vi "readParameterFromXML.vi"(8 "error in (no error)":errorcluster, 10 "eventXML":refnum<k20>, 11 "ScriptEvent in":refnum<class "ScriptEvent.lvclass">) -> (0 "error out":errorcluster, 2 "eventXML out":refnum<k20>, 3 "ScriptEvent out":refnum<class "ScriptEvent.lvclass">)   [LabVIEW 2009, in "Tools.lvlib" / "Scripting.lvlib" / "ScriptEvent.lvclass"]
uses:
  ScriptEvent.lvclass
  <vilib>/xml/Close Reference(Node).vi
  ScriptEvent.lvclass/ScriptEvent.ctl
  <vilib>/xml/NI_XML.lvlib
  Program Files/National Instruments/LabVIEW 2009/resource/objmgr/DOMUserDefRef.rc
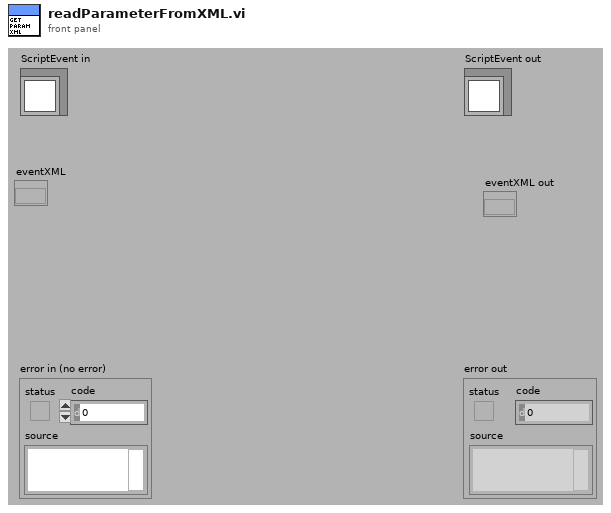
[diagram p1: front panel]
types:
  T1 = cluster{"parameter_name":string, "parameter_value":string, "type":enum16{"time", "time_difference", "value", "frequency", "phase", "ramp_time", "value_step", "time_step", "number_of_steps", "start_value", "end_value", "start_freq", "start_amp", "start_phase", "end_freq", "end_amp", "end_phase"}}
  T2 = enum16{"time", "time_difference", "value", "frequency", "phase", "ramp_time", "value_step", "time_step", "number_of_steps", "start_value", "end_value", "start_freq", "start_amp", "start_phase", "end_freq", "end_amp", "end_phase"}
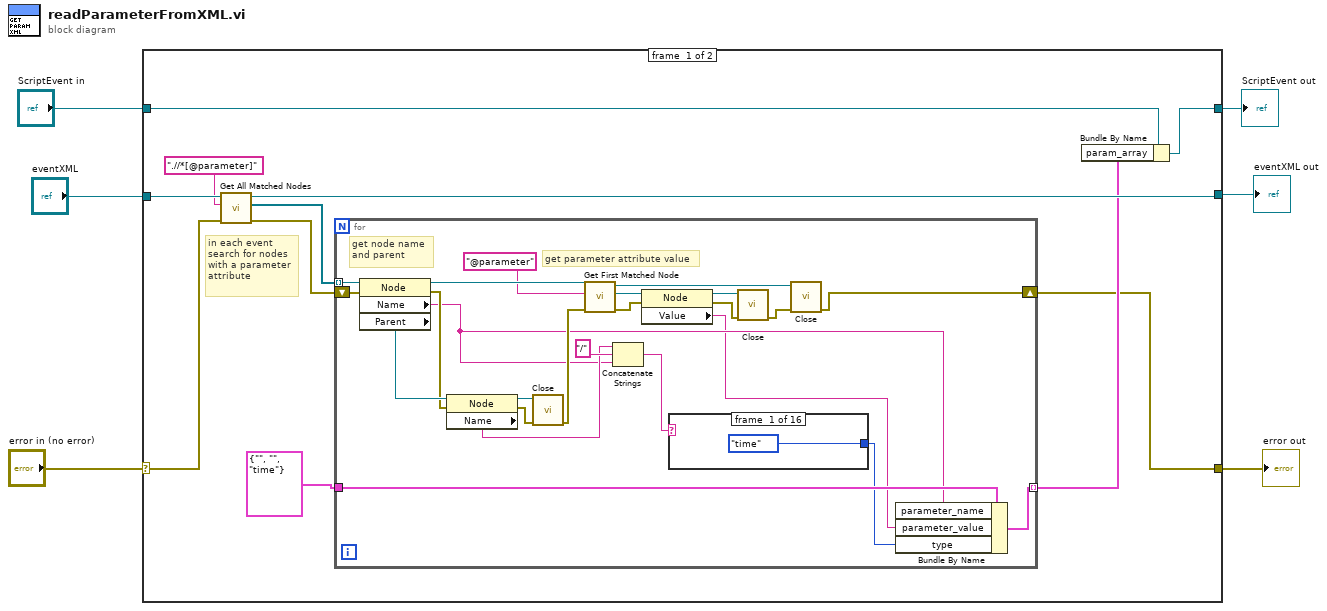
[diagram p0: block diagram]
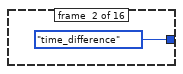
[diagram p2: hidden frame]
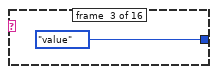
[diagram p3: hidden frame]
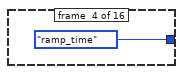
[diagram p4: hidden frame]
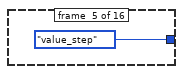
[diagram p5: hidden frame]
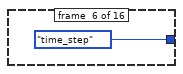
[diagram p6: hidden frame]
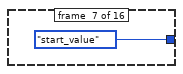
[diagram p7: hidden frame]
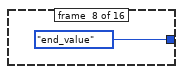
[diagram p8: hidden frame]
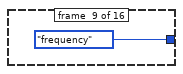
[diagram p9: hidden frame]
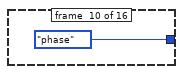
[diagram p10: hidden frame]
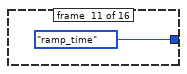
[diagram p11: hidden frame]
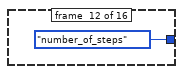
[diagram p12: hidden frame]
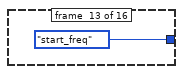
[diagram p13: hidden frame]
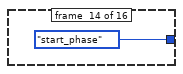
[diagram p14: hidden frame]
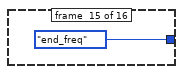
[diagram p15: hidden frame]
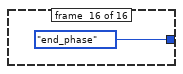
[diagram p16: hidden frame]
diagram:
  n1 = case shown="No Error" "error in (no error)" {
    selector: "error in (no error)" -> [w14 w59]
    tunnel: [w7 w59] -> w5
    tunnel: [w12 w58] -> w3
    tunnel: "ScriptEvent in" -> [w13 w58]
    tunnel: "eventXML" -> [w17 _]
    tunnel: [w16 _] -> w1
    frame #0 {
      # "in each event\nsearch for nodes\nwith a parameter\nattribute"
      n2 = call <vilib>:"Get All Matched Nodes.vi"("error in (no error)"=w14, "XPath expression"=".//*[@parameter]", "node in"=w17) -> ("error out"=w9:errorcluster, "node result array"=w11:refnum<k20>[], "node out"=w16:refnum<k20>)  [unwired: 6 in]
      n3 = for {
        shift-right: [w40] -> w7
        shift-left: w9 -> [w41]
        tunnel: T1 {"parameter_name"="", "parameter_value"="", "type"=enum."time"} ("param") -> [w23]
        tunnel: [w19] -> w8 mode=indexing
        tunnel: w11 -> [w18] mode=indexing
        # "get parameter attribute value"
        # "get node name\nand parent"
        n4 = property class="Node"(reference=w18, error in=w41) -> (reference out=w39:refnum<k20>, error out=w29:errorcluster, "Name"=w22:string, "Parent"=w30:refnum<k20>)
        n5 = property class="Node"(reference=w30, error in=w29) -> (reference out=w27:refnum<k20>, error out=w28:errorcluster, "Name"=w25:string)
        n6 = call-poly <vilib>:"Close.vi"("error in (no error)"=w28, "node"=w27) -> ("error out"=w26:errorcluster)  [unwired: 7 in]
        n7 = call <vilib>:"Get First Matched Node.vi"("error in (no error)"=w26, "XPath expression"="@parameter" ("search 2"), "node in"=w39) -> ("error out"=w36:errorcluster, "node result"=w37:refnum<k20>, "node out"=w32:refnum<k20>)  [unwired: 6 in]
        n8 = Concatenate Strings(w25, "/", w22) -> (w24:string)
        n9 = property class="Node"(reference=w37, error in=w36) -> (reference out=w35:refnum<k20>, error out=w34:errorcluster, "Value"=w21:string)
        n10 = case shown="\"stop/phase\"" w24 {
          tunnel: [T2."time" T2."time_difference" T2."value" T2."ramp_time" T2."value_step" T2."time_step" T2."start_value" T2."end_value" T2."frequency" T2."phase" T2."ramp_time" T2."number_of_steps" T2."start_freq" T2."start_phase" T2."end_freq" T2."end_phase"] -> w20
          frame #0 {
          }
          frame #1 {
          }
          frame #2 {
          }
          frame #3 {
          }
          frame #4 {
          }
          frame #5 {
          }
          frame #6 {
          }
          frame #7 {
          }
          frame #8 {
          }
          frame #9 {
          }
          frame #10 {
          }
          frame #11 {
          }
          frame #12 {
          }
          frame #13 {
          }
          frame #14 {
          }
          frame #15 {
          }
        }
        n11 = call-poly <vilib>:"Close.vi"("error in (no error)"=w34, "node"=w35) -> ("error out"=w33:errorcluster)  [unwired: 7 in]
        n12 = call-poly <vilib>:"Close.vi"("error in (no error)"=w33, "node"=w32) -> ("error out"=w40:errorcluster)  [unwired: 7 in]
        n13 = Bundle By Name(cluster=w23, "parameter_name"=w22, "parameter_value"=w21, "type"=w20) -> (w19:T1)
      }
      n14 = Bundle By Name(cluster=w13, "param_array"=w8) -> (w12:refnum<class "ScriptEvent.lvclass">)
    }
    frame #1 {
    }
  }
  "error out" <- w5
  "ScriptEvent out" <- w3
  "eventXML out" <- w1
